vi "prepractica 3.vi"() -> ()   [LabVIEW 2015]
uses:
  <vilib>/Analysis/Matrix/NI_Matrix.lvlib
  <vilib>/Analysis/Matrix/Numeric/Conversions/Array To Matrix - RA2.vi
panel:
  out "Si es divisible para 9":bool
  out "No es divisible para 9":bool
  in  "Numeric 2":dbl
  out "Si es primo":bool
  out "No es primo":bool
  in  "Numero a verificar:":dbl
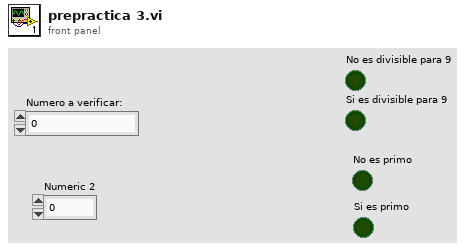
[diagram p1: front panel]
types:
  T1 = typedef "NI_Matrix.lvlib/RealMatrix.ctl" = dbl[][]
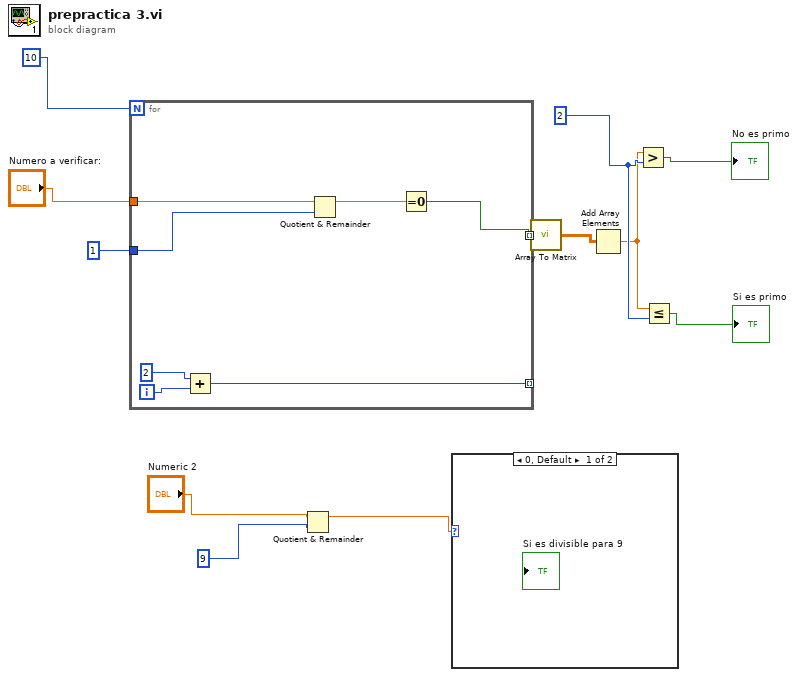
[diagram p0: block diagram]
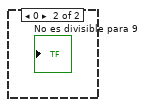
[diagram p2: hidden frame]
diagram:
  w8 = 2
  n1 = for {
    N: 10 -> [_]
    tunnel: [w16] -> _ mode=indexing
    tunnel: 1 -> [w15]
    tunnel: "Numero a verificar:" -> [w14]
    tunnel: [w12] -> _ mode=indexing
    i -> [w18]
    n2 = Add(x=2, y=w18) -> (x+y=w16:i32)
    n3 = Quotient & Remainder(x=w14, y=w15) -> (x-y*floor(x/y)=w13:dbl)  [unwired: 1 out]
    n4 = Equal To 0?(x=w13) -> (x = 0?=w12:bool)
  }
  n5 = Quotient & Remainder(x="Numeric 2", y=9) -> (x-y*floor(x/y)=w1:dbl)  [unwired: 1 out]
  n6 = case shown="0, Default" w1 {
    frame 0, Default {
    }
    frame 0 {
    }
  }
  n7 = call-poly <vilib>:"Array To Matrix.vi"() -> ("Real Matrix"=w4:T1)  [unwired: 1 in]
  n8 = Add Array Elements(numeric array=w4) -> (sum=w7:dbl)
  n9 = Greater?(x=w7, y=w8) -> (0:→"No es primo":bool)
  n10 = Less Or Equal?(x=w7, y=w8) -> (x <= y?=→"Si es primo":bool)
